vi "Read back eight integers from file.vi"(0 "File Path":path, 11 "error in (no error)":errorcluster) -> (2 "item 1":i32, 3 "item 2":i32, 4 "item 3":i32, 6 "item 4":i32, 8 "item 5":i32, 10 "item 6":i32, 13 "item 8":i32, 14 "item 7":i32, 15 "error out":errorcluster)   [LabVIEW 2013]
uses:
  <vilib>/Utility/file.llb/Read From Spreadsheet File (string).vi
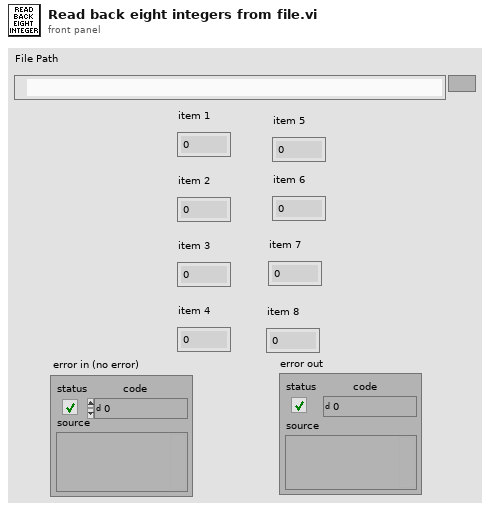
[diagram p1: front panel]
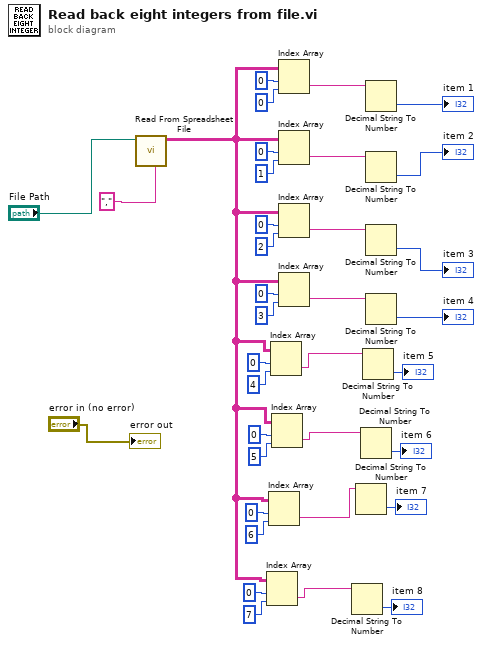
[diagram p0: block diagram]
diagram:
  n1 = call-poly <vilib>:"Read From Spreadsheet File.vi"("delimiter (\\t)"="," ("delimiter (\\t)"), "file path (dialog if empty)"="File Path") -> ("all rows"=w10:string[][])  [unwired: 5 in, 4 out]
  n2 = Index Array(array=w10, index (row)=0, index (col)=7 ("disabled index (col)")) -> (element=w6:string)
  n3 = Index Array(array=w10, index (row)=0, index (col)=6 ("disabled index (col)")) -> (element=w7:string)
  n4 = Index Array(array=w10, index (row)=0, index (col)=4 ("disabled index (col)")) -> (element=w9:string)
  n5 = Index Array(array=w10, index (row)=0, index (col)=5 ("disabled index (col)")) -> (element=w8:string)
  n6 = Index Array(array=w10, index (row)=0, index (col)=0 ("disabled index (col)")) -> (element=w29:string)
  n7 = Index Array(array=w10, index (row)=0, index (col)=1 ("disabled index (col)")) -> (element=w35:string)
  n8 = Index Array(array=w10, index (row)=0, index (col)=2 ("disabled index (col)")) -> (element=w31:string)
  n9 = Index Array(array=w10, index (row)=0, index (col)=3 ("disabled index (col)")) -> (element=w33:string)
  n10 = Decimal String To Number(string=w6) -> (number=→"item 8":i32)  [unwired: 2 in, 1 out]
  n11 = Decimal String To Number(string=w7) -> (number=→"item 7":i32)  [unwired: 2 in, 1 out]
  n12 = Decimal String To Number(string=w8) -> (number=→"item 6":i32)  [unwired: 2 in, 1 out]
  n13 = Decimal String To Number(string=w9) -> (number=→"item 5":i32)  [unwired: 2 in, 1 out]
  n14 = Decimal String To Number(string=w29) -> (number=→"item 1":i32)  [unwired: 2 in, 1 out]
  n15 = Decimal String To Number(string=w35) -> (number=→"item 2":i32)  [unwired: 2 in, 1 out]
  n16 = Decimal String To Number(string=w31) -> (number=→"item 3":i32)  [unwired: 2 in, 1 out]
  n17 = Decimal String To Number(string=w33) -> (number=→"item 4":i32)  [unwired: 2 in, 1 out]
  "error out" <- "error in (no error)"
